vi "SUB_SendAudo_TEST.vi"() -> ()   [LabVIEW 2011]
uses:
  <vilib>/Analysis/NI_AALBase.lvlib
  <vilib>/addons/Sound and Vibration/svt_Subset FFT/SVT Power Spectrum Subset (1 Ch).vi
  <vilib>/addons/Sound and Vibration/svt_Distortion/SVT THD and Harmonic Components (Time) (1 Ch).vi
  <vilib>/addons/Sound and Vibration/svt_Level/SoundVib_VibrationLevel.lvlib
  <vilib>/addons/Sound and Vibration/svt_Level/SVL Running RMS Level (1 Ch).vi
panel:
  out "THD":dbl format="%.2f"
  out "running RMS level [EU rms] 2":dbl=nan format="%.2f"
  out "running RMS level [EU rms]":dbl=nan format="%.2f"
  out "detected fundamental\nfrequency [Hz]":dbl format="%.2f"
  out "detected fundamental\namplitude":dbl format="%.2f"
  out "Waveform Graph":cluster{"f0":dbl, "df":dbl, "magnitude":dbl[]}(graph)
  out "Waveform Chart":dbl[](graph)
  in  "AO Amplitude (V)":dbl=0.1
  in  "Frequency (Hz)":dbl=1000.0
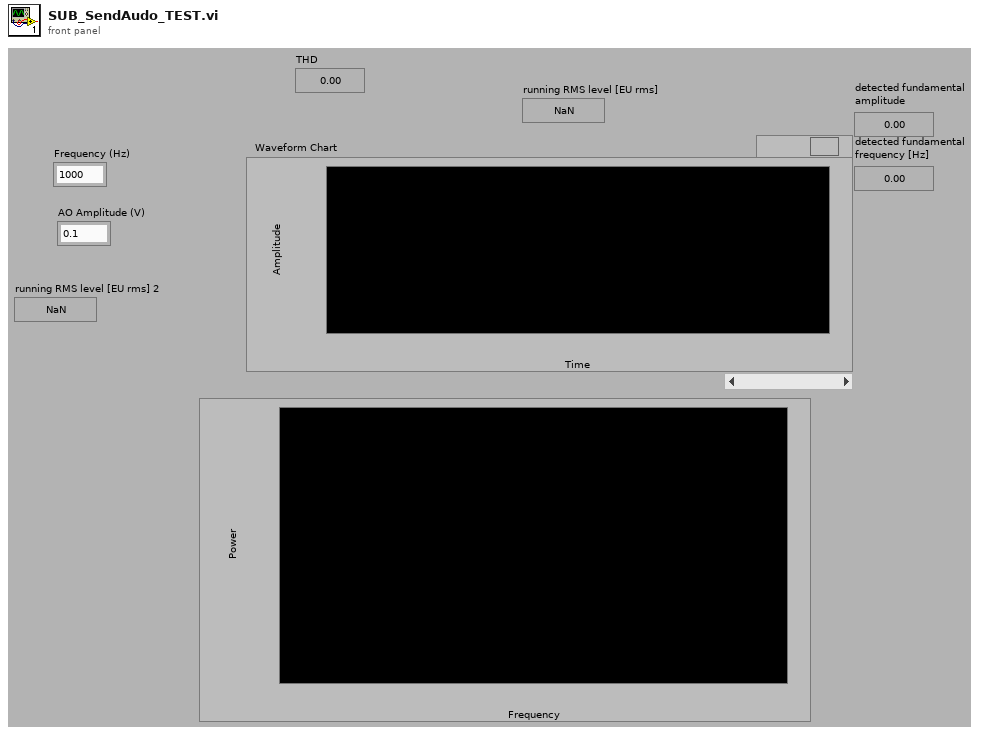
[diagram p1: front panel]
types:
  T1 = cluster{"THD units":enum16{"dB", "linear ratio", "%"}, "harmonic component amplitude units":enum16{"EU rms", "EU peak", "EU peak-peak", "dB ref fund"}, "detected fundamental amplitude units":enum16{"EU rms", "EU peak", "EU peak-peak"}}
  T2 = cluster{"THD+N units":enum16{"dB", "linear ratio", "%"}, "detected fundamental amplitude units":enum16{"EU rms", "EU peak", "EU peak-peak"}}
  T3 = cluster{"start frequency":dbl, "stop frequency":dbl}
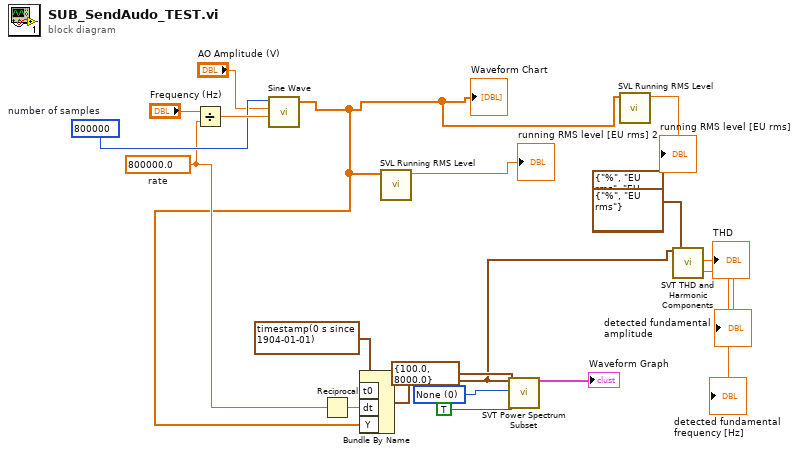
[diagram p0: block diagram]
diagram:
  (unwired) T2 {"THD+N units"=enum."%", "detected fundamental amplitude units"=enum."EU rms"} ("desired units")
  w12 = u16 0 items=["None ", "Hanning", "Hamming", "Blackman-Harris", "Exact Blackman", "Blackman", "Flat Top", "4 Term B-Harris ", "7 Term B-Harris", "Low Sidelobe"] ("window")
  w9 = 800000.0  # rate
  w17 = 800000  # number of samples
  n1 = Divide(x="Frequency (Hz)", y=w9) -> (x/y=w19:dbl)
  n2 = call <vilib>:"Sine Wave.vi"("samples"=w17, "amplitude"="AO Amplitude (V)", "frequency"=w19) -> ("sine wave"=w3:dbl[])  [unwired: 2 in, 2 out]
  "Waveform Chart" <- w3
  n3 = Reciprocal(x=w9) -> (1/x=w15:dbl)
  n4 = Bundle By Name("t0"=timestamp(0 s since 1904-01-01), "dt"=w15, "Y"=w3) -> (w8:waveform(dbl))  [unwired: 1 in]
  n5 = call-poly <vilib>:"SVL Running RMS Level.vi"("scaled signal [EU]"=w3) -> ("running RMS level [EU rms]"=→"running RMS level [EU rms] 2":dbl)  [unwired: 7 in, 3 out]
  n6 = call-poly <vilib>:"SVT Power Spectrum Subset.vi"("scaled signal [EU]"=w8, "window"=w12, "frequency range"=T3 {"start frequency"=100.0, "stop frequency"=8000.0}, "dB On (T)"=TRUE) -> ("power spectrum [dB EU]"=→"Waveform Graph":cluster{"f0":dbl, "df":dbl, "magnitude":dbl[]})  [unwired: 10 in, 5 out]
  n7 = call-poly <vilib>:"SVL Running RMS Level.vi"("scaled signal [EU]"=w3) -> ("running RMS level [EU rms]"=→"running RMS level [EU rms]":dbl)  [unwired: 7 in, 3 out]
  n8 = call-poly <vilib>:"SVT THD and Harmonic Components.vi"("scaled signal [EU]"=w8, "desired units"=T1 {"THD units"=enum."%", "harmonic component amplitude units"=enum."EU rms", "detected fundamental amplitude units"=enum."EU rms"}) -> ("detected fundamental\nfrequency [Hz]"=→"detected fundamental\nfrequency [Hz]":dbl, "detected fundamental\namplitude"=→"detected fundamental\namplitude":dbl, "THD"=→"THD":dbl)  [unwired: 10 in, 5 out]
